vi "Create Send Method.vi"(7 "AppInst":refnum<vi>, 8 "error in (no error)":errorcluster, 9 "Target Method":string="Change", 10 "New Class":path) -> (0 "error out":errorcluster, 1 "New Send Method":path)   [LabVIEW 2020, in "Message Maker.lvlib"]
uses:
  Message Maker.lvlib
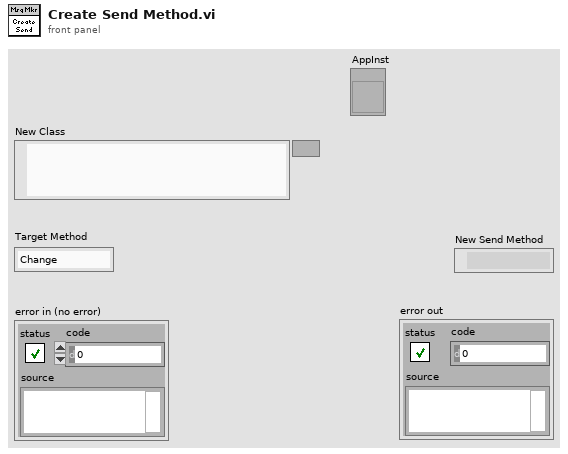
[diagram p1: front panel]
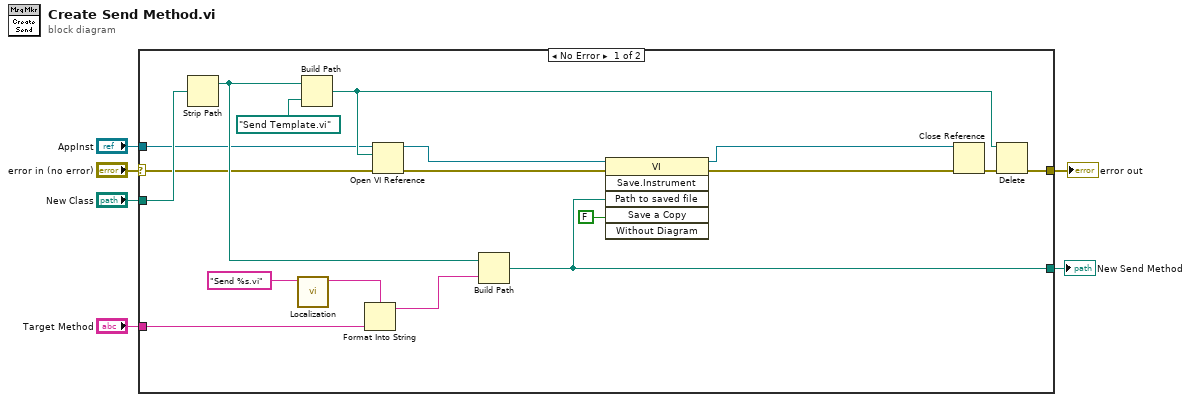
[diagram p0: block diagram]
diagram:
  n1 = case shown="No Error" "error in (no error)" {
    selector: "error in (no error)" -> [w10 w25]
    tunnel: [w21 _] -> w6
    tunnel: "Target Method" -> [w19 _]
    tunnel: [w17 w25] -> w4
    tunnel: "New Class" -> [w14 _]
    tunnel: "AppInst" -> [w9 _]
    frame No Error {
      n2 = Strip Path(path=w14) -> (stripped path=w15:path)  [unwired: 1 out]
      n3 = call "Localization.vi"("Unlocalized"="Send %s.vi") -> ("Localized"=w12:string)  [unwired: 10 in]
      n4 = Build Path(base path=w15, name or relative path=path "Send Template.vi") -> (appended path=w20:path)
      n5 = Format Into String(format string=w12, w19) -> (resulting string=w24:string)  [unwired: 2 in, 1 out]
      n6 = Open VI Reference(application reference (local)=w9, vi path=w20, error in (no error)=w10) -> (vi reference=w13:refnum<vi>, error out=w18:errorcluster)  [unwired: 3 in]
      n7 = Build Path(base path=w15, name or relative path=w24) -> (appended path=w21:path)
      n8 = invoke class="VI" method="Save.Instrument"(reference=w13, error in=w18, "Path to saved file"=w21, "Save a Copy"=FALSE) -> (reference out=w8:refnum<vi>, error out=w7:errorcluster)  [unwired: 2 in, 4 out]
      n9 = Close Reference(reference=w8, error in (no error)=w7) -> (error out=w22:errorcluster)
      n10 = Delete(path (use dialog)=w20, error in=w22) -> (error out=w17:errorcluster)  [unwired: 3 in, 2 out]
    }
    frame Error {
    }
  }
  "error out" <- w4
  "New Send Method" <- w6
